vi "Data Streaming.vi"() -> ()   [LabVIEW 2019]
doc: "This VI creates two queues to pass data between parallel loops. Queues are most useful when you need to send data from one or more data sources to one data sink with no potential loss of data."
panel:
  out "Elements in queue":i32(slide) scale=0.0..10.0
  in  "Receiving Loop timing":u32=500
  out "Received Data":dbl(graph)
  out "Receiving Loop Iteration":i32
  out "Generation Loop Iteration":i32
  out "Timeout?":bool
  in  "Enqueue timeout (ms)":i32=-1
  out "Generated Data":dbl(graph)
  in  "Stop":bool
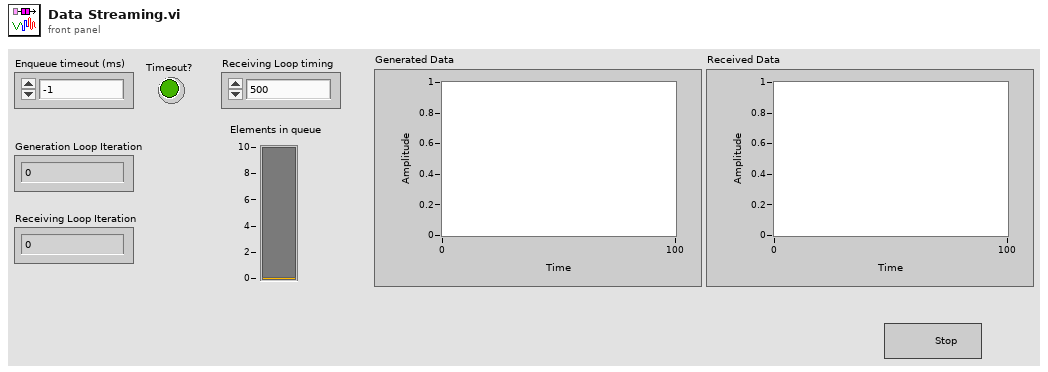
[diagram p1: front panel]
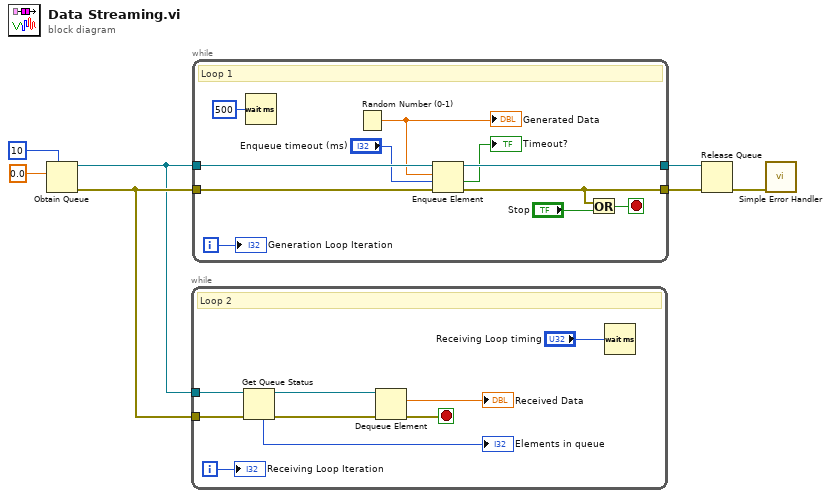
[diagram p0: block diagram]
diagram:
  n1 = Obtain Queue(max queue size (-1, unlimited)=10, element data type=0.0) -> (queue out=w1:refnum<queue>, error out=w2:errorcluster)  [unwired: 3 in, 1 out]
  n2 = while {
    tunnel: w2 -> [w15]
    tunnel: w1 -> [w14]
    i -> [w16]
    stop <- w11 stop-if-true
    # "Loop 2"
    n3 = Get Queue Status(queue=w14, error in (no error)=w15) -> (queue out=w13:refnum<queue>, error out=w12:errorcluster, # elements in queue=→"Elements in queue":i32)  [unwired: 1 in, 5 out]
    n4 = Dequeue Element(queue=w13, error in (no error)=w12) -> (element=→"Received Data":dbl, error out=w11:errorcluster)  [unwired: 1 in, 2 out]
    n5 = Wait (ms)(milliseconds to wait="Receiving Loop timing") -> ()  [unwired: 1 out]
    "Receiving Loop Iteration" <- w16
  }
  n6 = while {
    tunnel: w2 -> [w26]
    tunnel: w1 -> [w25]
    tunnel: [w24] -> w5
    tunnel: [w22] -> w6
    i -> [w17]
    stop <- w20 stop-if-true
    # "Loop 1"
    n7 = Wait (ms)(milliseconds to wait=u32 500) -> ()  [unwired: 1 out]
    n8 = Random Number (0-1)() -> (number: 0 to 1=w23:dbl)
    "Generated Data" <- w23
    n9 = Enqueue Element(queue=w25, element=w23, timeout in ms (-1)="Enqueue timeout (ms)", error in (no error)=w26) -> (queue out=w24:refnum<queue>, timed out?=→"Timeout?":bool, error out=w22:errorcluster)
    n10 = Or(x=w22, y="Stop") -> (x .or. y?=w20:bool)
    "Generation Loop Iteration" <- w17
  }
  n11 = Release Queue(queue=w5, error in (no error)=w6) -> (error out=w4:errorcluster)  [unwired: 1 in, 2 out]
  n12 = call <vilib>:"Simple Error Handler.vi"("error in (no error)"=w4) -> ()  [unwired: 4 in, 5 out]
